vi "Wait for Operation Complete.vi"(8 "error in (no error)":errorcluster, 9 "Maximum Time (10000ms)":u32=10000, 11 "VISA resource name":refnum<visa-resource-name>) -> (0 "error out":errorcluster, 3 "VISA resource name out":refnum<visa-resource-name>)   [LabVIEW 2009, in "Tektronix DPO MSO 2000 4000 Series.lvlib"]
doc: "This VI waits for the instrument to complete the execution of all pending operations. The <B>Timeout</B> control specifies the maximum time to wait for operation complete in milliseconds."
uses:
  <instrlib>/Tektronix DPO MSO 2000 4000 Series/Tektronix DPO MSO 2000 4000 Series.lvlib
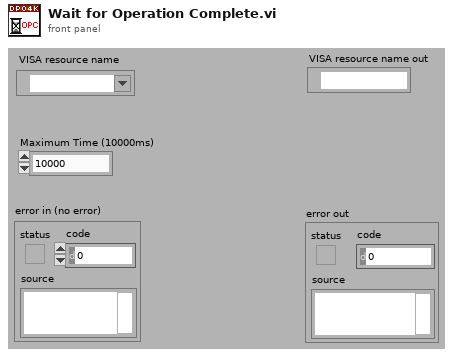
[diagram p1: front panel]
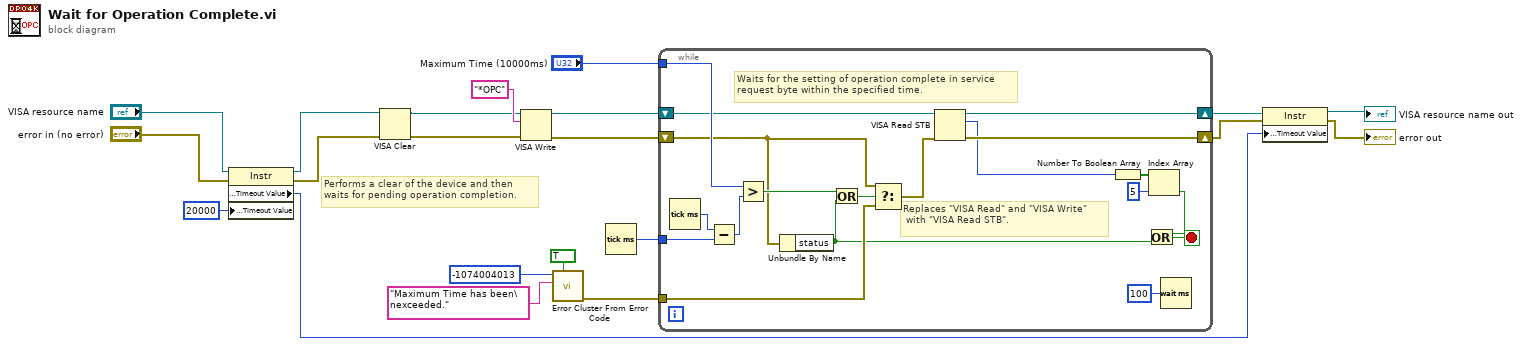
[diagram p0: block diagram]
diagram:
  # "Performs a clear of the device and then\nwaits for pending operation completion."
  n1 = property class="Instr"(reference="VISA resource name", error in="error in (no error)", "General Settings:Timeout Value"=u32 20000) -> (reference out=w12:refnum<visa-resource-name>, error out=w11:errorcluster, "General Settings:Timeout Value"=w9:u32)
  n2 = VISA Clear(VISA resource name=w12, error in (no error)=w11) -> (VISA resource name out=w2:refnum<visa-resource-name>, error out=w1:errorcluster)
  n3 = VISA Write(VISA resource name=w2, write buffer="*OPC", error in (no error)=w1) -> (VISA resource name out=w18:refnum<visa-resource-name>, error out=w17:errorcluster)  [unwired: 1 out]
  n4 = call <vilib>:"Error Cluster From Error Code.vi"("show call chain? (False)"=TRUE, "error message (\"\")"="Maximum Time has been\nexceeded." ("error message (\"\")"), "error code (0)"=-1074004013) -> ("error out"=w16:errorcluster)  [unwired: 6 in]
  n5 = Tick Count (ms)() -> (millisecond timer value=w20:u32)
  n6 = while {
    tunnel: w20 -> [w37]
    tunnel: "Maximum Time (10000ms)" -> [w35]
    shift-right: [w24] -> w8
    shift-left: w18 -> [w27]
    shift-right: [w25] -> w7
    shift-left: w17 -> [w26]
    tunnel: w16 -> [w33]
    stop <- w32 stop-if-true
    # "Replaces \"VISA Read\" and \"VISA Write\"\n with \"VISA Read STB\"."
    # "Waits for the setting of operation complete in service\nrequest byte within the specified time."
    n7 = Tick Count (ms)() -> (millisecond timer value=w38:u32)
    n8 = Subtract(x=w38, y=w37) -> (x-y=w36:u32)
    n9 = Greater?(x=w35, y=w36) -> (0:w30:bool)
    n10 = Unbundle By Name(w26) -> ("status"=w29:bool)
    n11 = Or(x=w30, y=w29) -> (x .or. y?=w34:bool)
    n12 = Select(t=w26, s=w34, f=w33) -> (s? t:f=w22:errorcluster)
    n13 = VISA Read STB(8:w22, 11:w27) -> (0:w25:errorcluster, 2:w23:u16, 3:w24:refnum<visa-resource-name>)
    n14 = Number To Boolean Array(number=w23) -> (Boolean array=w40:bool[])
    n15 = Index Array(array=w40, index=5) -> (element=w31:bool)
    n16 = Or(x=w31, y=w29) -> (x .or. y?=w32:bool)
    n17 = Wait (ms)(milliseconds to wait=u32 100) -> ()  [unwired: 1 out]
  }
  n18 = property class="Instr"(reference=w8, error in=w7, "General Settings:Timeout Value"=w9) -> (reference out=→"VISA resource name out":refnum<visa-resource-name>, error out=→"error out":errorcluster)
